vi "BLE_Request_Connect.vi"(0 ".NET Refnum in":refnum<k24>, 5 "BluetoothAddress":u64, 11 "error in (no error)":errorcluster) -> (4 ".NET Refnum out":refnum<k24>, 6 "ConnectBLE":string, 15 "error out":errorcluster)   [LabVIEW 2020, in "BLE.lvlib"]
uses:
  C:/Users/Trait/Desktop/LabView Project/LabView BLE DataACQ/BLELib.dll
  BLELib.dll
  BLE.lvlib
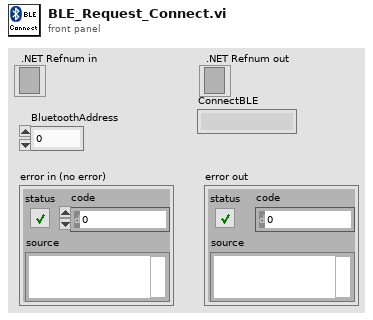
[diagram p1: front panel]
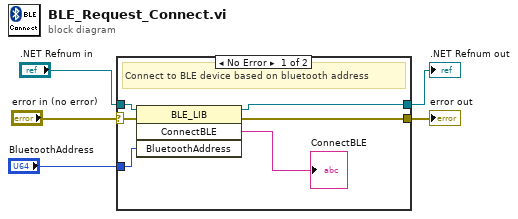
[diagram p0: block diagram]
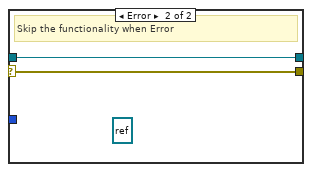
[diagram p2: hidden frame]
diagram:
  n1 = case shown="No Error" "error in (no error)" {
    selector: "error in (no error)" -> [w8 w12]
    tunnel: "BluetoothAddress" -> [w11 _]
    tunnel: [w10 w12] -> w4
    tunnel: ".NET Refnum in" -> [w9 w13]
    tunnel: [w7 w13] -> w2
    frame No Error {
      # "Connect to BLE device based on bluetooth address"
      n2 = invoke class="BLE_LIB" method="ConnectBLE"(reference=w9, error in=w8, "BluetoothAddress"=w11) -> (reference out=w7:refnum<k24>, error out=w10:errorcluster, "ConnectBLE"=→"ConnectBLE":string)  [unwired: 1 in, 1 out]
    }
    frame Error {
      (unwired) refnum<k24> refnum ("ConnectBLE")
      # "Skip the functionality when Error"
    }
  }
  "error out" <- w4
  ".NET Refnum out" <- w2
